vi "Get Test Executive Version.vi"(7 "Unique ID":string, 8 "error in (no error)":errorcluster, 11 "Test Executive in":refnum<class "Test Executive.lvclass">) -> (0 "error out":errorcluster, 1 "Found?":bool, 2 "Test Exec Version":string, 3 "Test Executive out":refnum<class "Test Executive.lvclass">)   [LabVIEW 2017, in "Test Executive.lvlib" / "Test Executive.lvclass"]
uses:
  <vilib>/gpm_packages/@cs/test-executive/Source/Test Executive/TestExecutive/Test Executive.lvclass
  <vilib>/gpm_packages/@cs/test-executive/Source/Test Executive/TestExecutive/Test Executive.lvclass/Test Executive.ctl
  <vilib>/gpm_packages/@cs/linked-list/Source/Linked List/Linked List Ref/Linked List Ref.lvclass
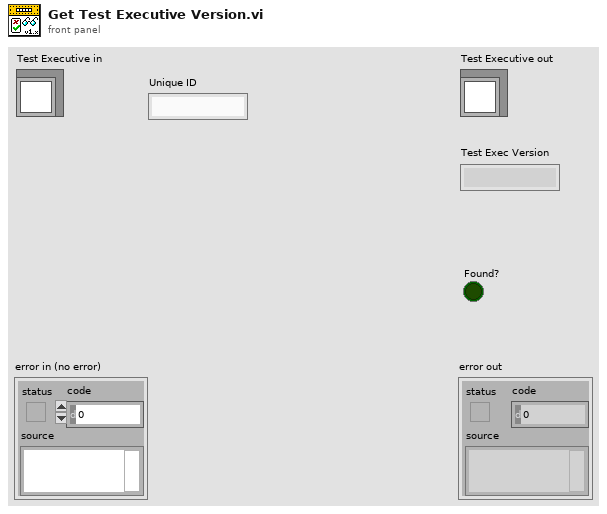
[diagram p1: front panel]
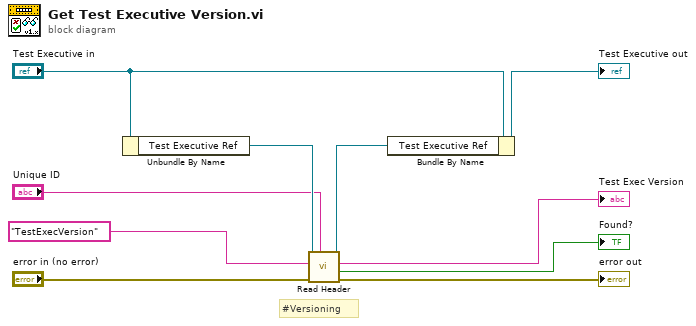
[diagram p0: block diagram]
diagram:
  # "#Versioning"
  n1 = Unbundle By Name("Test Executive in") -> ("Test Executive Ref"=w10:refnum<data-value>)
  n2 = call <vilib>:"Read Header.vi"("Linked List ID"="Unique ID", "error in (no error)"="error in (no error)", "Header Name"="TestExecVersion" ("String"), "Linked List Ref"=w10) -> ("error out"=→"error out":errorcluster, "found"=→"Found?":bool, "Header Value"=→"Test Exec Version":string, "Linked List Ref out"=w9:refnum<data-value>)  [unwired: 4 in]
  n3 = Bundle By Name(cluster="Test Executive in", "Test Executive Ref"=w9) -> (→"Test Executive out":refnum<class "Test Executive.lvclass">)
